vi "Numeric String to Bytes.vi"(9 "Type":T1(ring), 11 "String":string) -> (0 "error out":errorcluster, 3 "Byte Data":u8[](array[numeric]) format="%02x")   [LabVIEW 2020]
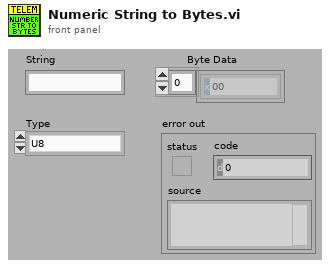
[diagram p1: front panel]
types:
  T1 = enum16{"U8", "U16", "U32", "U64", "I8", "I16", "I32", "I64"}
  T2 = cluster{"Byte Data[0]":u8, "Byte Data[1]":u8, "Byte Data[2]":u8, "Byte Data[3]":u8}
  T3 = cluster{"Byte Data[0]":u8, "Byte Data[1]":u8, "Byte Data[2]":u8, "Byte Data[3]":u8, "Byte Data[4]":u8, "Byte Data[5]":u8, "Byte Data[6]":u8, "Byte Data[7]":u8}
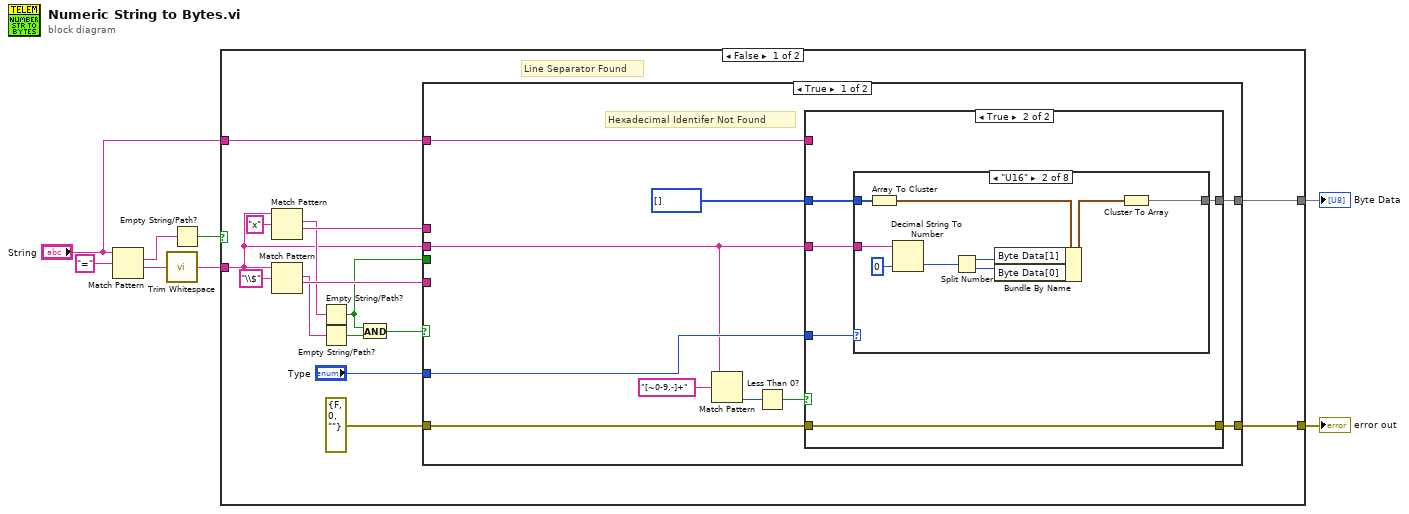
[diagram p0: block diagram]
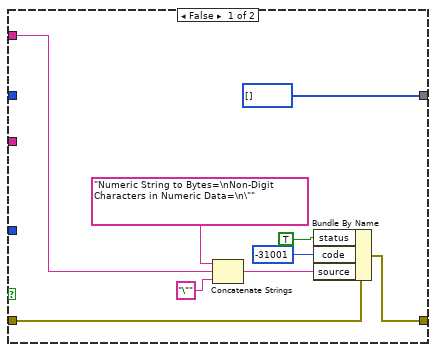
[diagram p2: hidden frame]
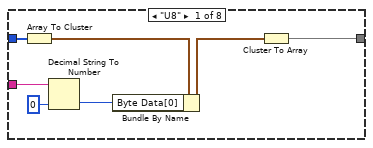
[diagram p3: hidden frame]
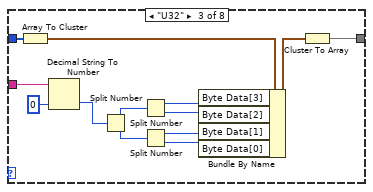
[diagram p4: hidden frame]
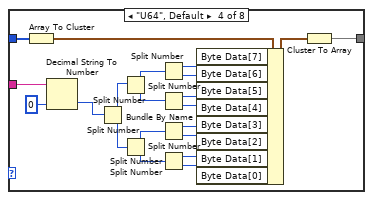
[diagram p5: hidden frame]
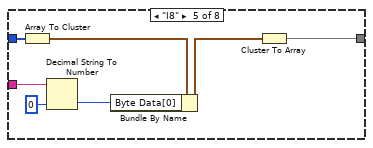
[diagram p6: hidden frame]
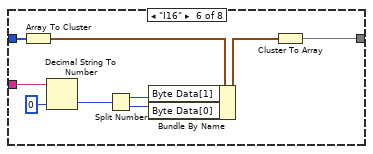
[diagram p7: hidden frame]
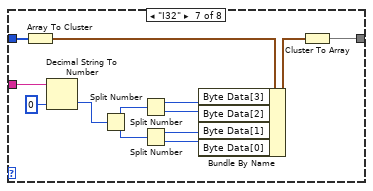
[diagram p8: hidden frame]
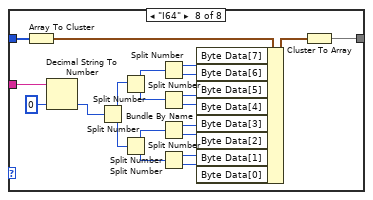
[diagram p9: hidden frame]
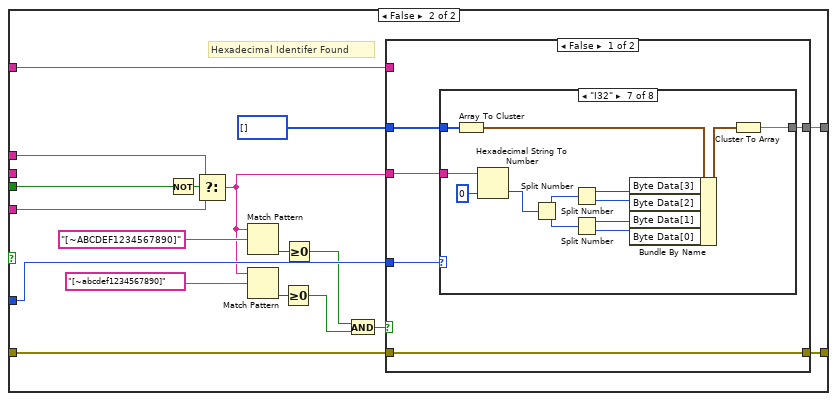
[diagram p10: hidden frame]
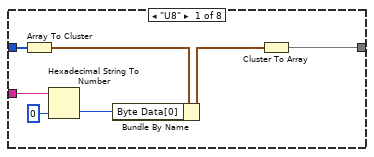
[diagram p11: hidden frame]
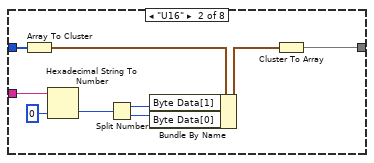
[diagram p12: hidden frame]
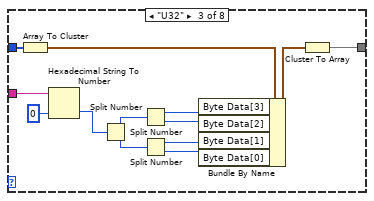
[diagram p13: hidden frame]
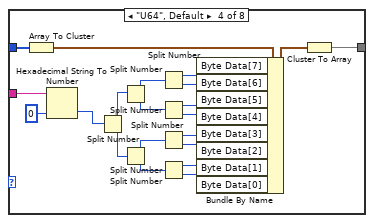
[diagram p14: hidden frame]
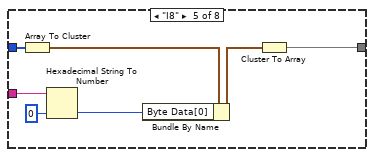
[diagram p15: hidden frame]
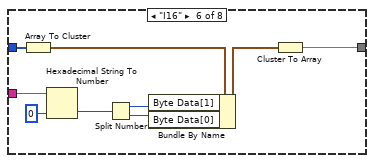
[diagram p16: hidden frame]
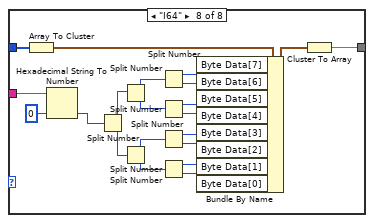
[diagram p17: hidden frame]
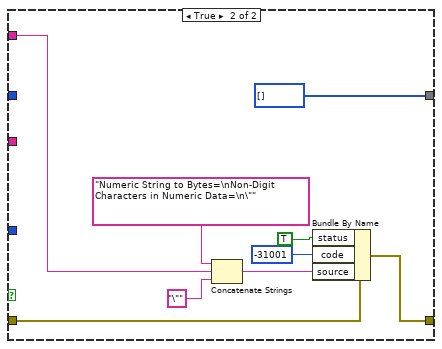
[diagram p18: hidden frame]
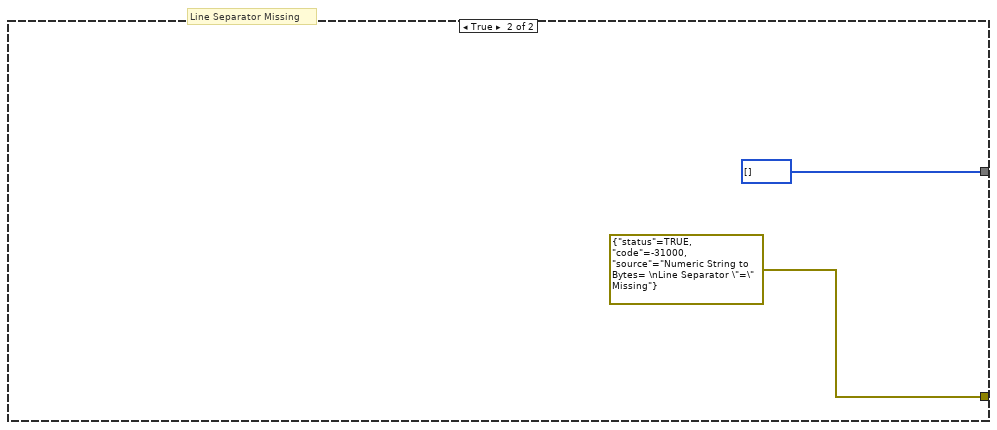
[diagram p19: hidden frame]
diagram:
  n1 = Match Pattern(string="String", regular expression="=") -> (match substring=w7:string, after substring=w6:string)  [unwired: 1 in, 2 out]
  n2 = call <vilib>:"Trim Whitespace.vi"("string"=w6) -> ("trimmed string"=w2:string)  [unwired: 1 in]
  n3 = Empty String/Path?(string/path=w7) -> (empty?=w5:bool)
  n4 = case shown="False" w5 {
    tunnel: w2 -> [w10 _]
    tunnel: [w13 u8[] [] ("Byte Data")] -> w4
    tunnel: [w11 errorcluster {"status"=TRUE, "code"=-31000, "source"="Numeric String to Bytes= \nLine Separator \"=\" Missing"} ("error out")] -> w3
    tunnel: "String" -> [w9 _]
    frame False {
      # "Line Separator Found"
      n5 = Match Pattern(string=w10, regular expression="x") -> (match substring=w19:string, after substring=w21:string)  [unwired: 1 in, 2 out]
      n6 = Match Pattern(string=w10, regular expression="\\$") -> (match substring=w18:string, after substring=w20:string)  [unwired: 1 in, 2 out]
      n7 = Empty String/Path?(string/path=w19) -> (empty?=w15:bool)
      n8 = Empty String/Path?(string/path=w18) -> (empty?=w16:bool)
      n9 = And(x=w15, y=w16) -> (x .and. y?=w17:bool)
      n10 = case shown="True" w17 {
        tunnel: w21 -> [_ w162]
        tunnel: w20 -> [_ w161]
        tunnel: w15 -> [_ w159]
        tunnel: [w31 w163] -> w13
        tunnel: w10 -> [w25 _]
        tunnel: "Type" -> [w33 w165]
        tunnel: errorcluster {"status"=FALSE, "code"=0, "source"=""} ("error out") -> [w29 w155]
        tunnel: [w30 w158] -> w11
        tunnel: w9 -> [w24 w150]
        frame True {
          # "Hexadecimal Identifer Not Found"
          n11 = Match Pattern(string=w25, regular expression="[~0-9,-]+") -> (offset past match=w27:i32)  [unwired: 1 in, 3 out]
          n12 = Less Than 0?(x=w27) -> (x < 0?=w26:bool)
          n13 = case shown="True" w26 {
            tunnel: w25 -> [_ w47]
            tunnel: w33 -> [_ w46]
            tunnel: u8[] [] ("Byte Data") -> [_ w45]
            tunnel: [u8[] [] ("Byte Data") w44] -> w31
            tunnel: [w36 w43] -> w30
            tunnel: w29 -> [w35 w43]
            tunnel: w24 -> [w34 _]
            frame False {
              n14 = Concatenate Strings("Numeric String to Bytes=\nNon-Digit Characters in Numeric Data=\n\"" ("source"), w34, "\"") -> (w37:string)
              n15 = Bundle By Name(cluster=w35, "status"=TRUE, "code"=-31001, "source"=w37) -> (w36:errorcluster)
            }
            frame True {
              n16 = case shown="\"U16\"" w46 {
                tunnel: w47 -> [w49 w57 w65 w97 w104 w113 w126 w147]
                tunnel: w45 -> [w50 w56 w68 w79 w102 w111 w124 w145]
                tunnel: [w48 w55 w69 w78 w98 w105 w114 w127] -> w44
                frame "U8" {
                  n17 = Array To Cluster(array=w50) -> (cluster=w53:cluster{"Byte Data[0]":u8})
                  n18 = Decimal String To Number(string=w49, default (0L)=u8 0 ("default (0 I32)")) -> (number=w52:u8)  [unwired: 1 in, 1 out]
                  n19 = Bundle By Name(cluster=w53, "Byte Data[0]"=w52) -> (w51:cluster{"Byte Data[0]":u8})
                  n20 = Cluster To Array(cluster=w51) -> (array=w48:u8[])
                }
                frame "U16" {
                  n21 = Array To Cluster(array=w56) -> (cluster=w62:cluster{"Byte Data[0]":u8, "Byte Data[1]":u8})
                  n22 = Decimal String To Number(string=w57, default (0L)=u16 0 ("default (0 I32)")) -> (number=w61:u16)  [unwired: 1 in, 1 out]
                  n23 = Split Number(x=w61) -> (hi(x)=w60:u8, lo(x)=w59:u8)
                  n24 = Bundle By Name(cluster=w62, "Byte Data[1]"=w60, "Byte Data[0]"=w59) -> (w58:cluster{"Byte Data[0]":u8, "Byte Data[1]":u8})
                  n25 = Cluster To Array(cluster=w58) -> (array=w55:u8[])
                }
                frame "U32" {
                  n26 = Array To Cluster(array=w68) -> (cluster=w67:T2)
                  n27 = Decimal String To Number(string=w65, default (0L)=u32 0 ("default (0 I32)")) -> (number=w64:u32)  [unwired: 1 in, 1 out]
                  n28 = Split Number(x=w64) -> (hi(x)=w75:u16, lo(x)=w76:u16)
                  n29 = Split Number(x=w75) -> (hi(x)=w74:u8, lo(x)=w73:u8)
                  n30 = Split Number(x=w76) -> (hi(x)=w72:u8, lo(x)=w71:u8)
                  n31 = Bundle By Name(cluster=w67, "Byte Data[3]"=w74, "Byte Data[2]"=w73, "Byte Data[1]"=w72, "Byte Data[0]"=w71) -> (w70:T2)
                  n32 = Cluster To Array(cluster=w70) -> (array=w69:u8[])
                }
                frame "U64", Default {
                  n33 = Array To Cluster(array=w79) -> (cluster=w95:T3)
                  n34 = Decimal String To Number(string=w97, default (0L)=u64 0 ("default (0 I32)")) -> (number=w77:u64)  [unwired: 1 in, 1 out]
                  n35 = Split Number(x=w77) -> (hi(x)=w94:u32, lo(x)=w93:u32)
                  n36 = Split Number(x=w94) -> (hi(x)=w91:u16, lo(x)=w92:u16)
                  n37 = Split Number(x=w93) -> (hi(x)=w90:u16, lo(x)=w89:u16)
                  n38 = Split Number(x=w91) -> (hi(x)=w88:u8, lo(x)=w87:u8)
                  n39 = Split Number(x=w92) -> (hi(x)=w86:u8, lo(x)=w85:u8)
                  n40 = Split Number(x=w90) -> (hi(x)=w84:u8, lo(x)=w83:u8)
                  n41 = Split Number(x=w89) -> (hi(x)=w82:u8, lo(x)=w81:u8)
                  n42 = Bundle By Name(cluster=w95, "Byte Data[7]"=w88, "Byte Data[6]"=w87, "Byte Data[5]"=w86, "Byte Data[4]"=w85, "Byte Data[3]"=w84, "Byte Data[2]"=w83, "Byte Data[1]"=w82, "Byte Data[0]"=w81) -> (w80:T3)
                  n43 = Cluster To Array(cluster=w80) -> (array=w78:u8[])
                }
                frame "I8" {
                  n44 = Array To Cluster(array=w102) -> (cluster=w101:cluster{"Byte Data[0]":u8})
                  n45 = Decimal String To Number(string=w104, default (0L)=i8 0 ("default (0 I32)")) -> (number=w100:i8)  [unwired: 1 in, 1 out]
                  n46 = Bundle By Name(cluster=w101, "Byte Data[0]"=w100) -> (w99:cluster{"Byte Data[0]":u8})
                  n47 = Cluster To Array(cluster=w99) -> (array=w98:u8[])
                }
                frame "I16" {
                  n48 = Array To Cluster(array=w111) -> (cluster=w110:cluster{"Byte Data[0]":u8, "Byte Data[1]":u8})
                  n49 = Decimal String To Number(string=w113, default (0L)=i16 0 ("default (0 I32)")) -> (number=w109:i16)  [unwired: 1 in, 1 out]
                  n50 = Split Number(x=w109) -> (hi(x)=w108:u8, lo(x)=w107:u8)
                  n51 = Bundle By Name(cluster=w110, "Byte Data[1]"=w108, "Byte Data[0]"=w107) -> (w106:cluster{"Byte Data[0]":u8, "Byte Data[1]":u8})
                  n52 = Cluster To Array(cluster=w106) -> (array=w105:u8[])
                }
                frame "I32" {
                  n53 = Array To Cluster(array=w124) -> (cluster=w123:T2)
                  n54 = Decimal String To Number(string=w126, default (0L)=0 ("default (0 I32)")) -> (number=w120:i32)  [unwired: 1 in, 1 out]
                  n55 = Split Number(x=w120) -> (hi(x)=w121:u16, lo(x)=w122:u16)
                  n56 = Split Number(x=w121) -> (hi(x)=w119:u8, lo(x)=w118:u8)
                  n57 = Split Number(x=w122) -> (hi(x)=w117:u8, lo(x)=w116:u8)
                  n58 = Bundle By Name(cluster=w123, "Byte Data[3]"=w119, "Byte Data[2]"=w118, "Byte Data[1]"=w117, "Byte Data[0]"=w116) -> (w115:T2)
                  n59 = Cluster To Array(cluster=w115) -> (array=w114:u8[])
                }
                frame "I64" {
                  n60 = Array To Cluster(array=w145) -> (cluster=w144:T3)
                  n61 = Decimal String To Number(string=w147, default (0L)=i64 0 ("default (0 I32)")) -> (number=w143:i64)  [unwired: 1 in, 1 out]
                  n62 = Split Number(x=w143) -> (hi(x)=w142:u32, lo(x)=w141:u32)
                  n63 = Split Number(x=w142) -> (hi(x)=w139:u16, lo(x)=w140:u16)
                  n64 = Split Number(x=w141) -> (hi(x)=w138:u16, lo(x)=w137:u16)
                  n65 = Split Number(x=w139) -> (hi(x)=w136:u8, lo(x)=w135:u8)
                  n66 = Split Number(x=w140) -> (hi(x)=w134:u8, lo(x)=w133:u8)
                  n67 = Split Number(x=w138) -> (hi(x)=w132:u8, lo(x)=w131:u8)
                  n68 = Split Number(x=w137) -> (hi(x)=w130:u8, lo(x)=w129:u8)
                  n69 = Bundle By Name(cluster=w144, "Byte Data[7]"=w136, "Byte Data[6]"=w135, "Byte Data[5]"=w134, "Byte Data[4]"=w133, "Byte Data[3]"=w132, "Byte Data[2]"=w131, "Byte Data[1]"=w130, "Byte Data[0]"=w129) -> (w128:T3)
                  n70 = Cluster To Array(cluster=w128) -> (array=w127:u8[])
                }
              }
            }
          }
        }
        frame False {
          # "Hexadecimal Identifer Found"
          n71 = Not(x=w159) -> (.not. x?=w160:bool)
          n72 = Select(t=w162, s=w160, f=w161) -> (s? t:f=w151:string)
          n73 = Match Pattern(string=w151, regular expression="[~ABCDEF1234567890]") -> (offset past match=w156:i32)  [unwired: 1 in, 3 out]
          n74 = Match Pattern(string=w151, regular expression="[~abcdef1234567890]") -> (offset past match=w152:i32)  [unwired: 1 in, 3 out]
          n75 = Greater Or Equal To 0?(x=w152) -> (x >= 0?=w148:bool)
          n76 = Greater Or Equal To 0?(x=w156) -> (x >= 0?=w154:bool)
          n77 = And(x=w154, y=w148) -> (x .and. y?=w153:bool)
          n78 = case shown="False" w153 {
            tunnel: w165 -> [w170 _]
            tunnel: u8[] [] ("Byte Data") -> [w169 _]
            tunnel: [w168 u8[] [] ("Byte Data")] -> w163
            tunnel: w151 -> [w167 _]
            tunnel: [w166 w277] -> w158
            tunnel: w155 -> [w166 w278]
            tunnel: w150 -> [_ w271]
            frame False {
              n79 = case shown="\"I32\"" w170 {
                tunnel: w167 -> [w172 w180 w188 w220 w227 w236 w249 w270]
                tunnel: w169 -> [w173 w179 w191 w202 w225 w234 w247 w268]
                tunnel: [w171 w178 w192 w201 w222 w228 w237 w250] -> w168
                frame "U8" {
                  n80 = Array To Cluster(array=w173) -> (cluster=w176:cluster{"Byte Data[0]":u8})
                  n81 = Hexadecimal String To Number(string=w172, default (0uL)=u8 0 ("default (0 I32)")) -> (number=w175:u8)  [unwired: 1 in, 1 out]
                  n82 = Bundle By Name(cluster=w176, "Byte Data[0]"=w175) -> (w174:cluster{"Byte Data[0]":u8})
                  n83 = Cluster To Array(cluster=w174) -> (array=w171:u8[])
                }
                frame "U16" {
                  n84 = Array To Cluster(array=w179) -> (cluster=w185:cluster{"Byte Data[0]":u8, "Byte Data[1]":u8})
                  n85 = Hexadecimal String To Number(string=w180, default (0uL)=u16 0 ("default (0 I32)")) -> (number=w184:u16)  [unwired: 1 in, 1 out]
                  n86 = Split Number(x=w184) -> (hi(x)=w183:u8, lo(x)=w182:u8)
                  n87 = Bundle By Name(cluster=w185, "Byte Data[1]"=w183, "Byte Data[0]"=w182) -> (w181:cluster{"Byte Data[0]":u8, "Byte Data[1]":u8})
                  n88 = Cluster To Array(cluster=w181) -> (array=w178:u8[])
                }
                frame "U32" {
                  n89 = Array To Cluster(array=w191) -> (cluster=w190:T2)
                  n90 = Hexadecimal String To Number(string=w188, default (0uL)=u32 0 ("default (0 I32)")) -> (number=w187:u32)  [unwired: 1 in, 1 out]
                  n91 = Split Number(x=w187) -> (hi(x)=w198:u16, lo(x)=w199:u16)
                  n92 = Split Number(x=w198) -> (hi(x)=w197:u8, lo(x)=w196:u8)
                  n93 = Split Number(x=w199) -> (hi(x)=w195:u8, lo(x)=w194:u8)
                  n94 = Bundle By Name(cluster=w190, "Byte Data[3]"=w197, "Byte Data[2]"=w196, "Byte Data[1]"=w195, "Byte Data[0]"=w194) -> (w193:T2)
                  n95 = Cluster To Array(cluster=w193) -> (array=w192:u8[])
                }
                frame "U64", Default {
                  n96 = Array To Cluster(array=w202) -> (cluster=w218:T3)
                  n97 = Hexadecimal String To Number(string=w220, default (0uL)=u64 0 ("default (0 I32)")) -> (number=w200:u64)  [unwired: 1 in, 1 out]
                  n98 = Split Number(x=w200) -> (hi(x)=w217:u32, lo(x)=w216:u32)
                  n99 = Split Number(x=w217) -> (hi(x)=w214:u16, lo(x)=w215:u16)
                  n100 = Split Number(x=w216) -> (hi(x)=w213:u16, lo(x)=w212:u16)
                  n101 = Split Number(x=w214) -> (hi(x)=w211:u8, lo(x)=w210:u8)
                  n102 = Split Number(x=w215) -> (hi(x)=w209:u8, lo(x)=w208:u8)
                  n103 = Split Number(x=w213) -> (hi(x)=w207:u8, lo(x)=w206:u8)
                  n104 = Split Number(x=w212) -> (hi(x)=w205:u8, lo(x)=w204:u8)
                  n105 = Bundle By Name(cluster=w218, "Byte Data[7]"=w211, "Byte Data[6]"=w210, "Byte Data[5]"=w209, "Byte Data[4]"=w208, "Byte Data[3]"=w207, "Byte Data[2]"=w206, "Byte Data[1]"=w205, "Byte Data[0]"=w204) -> (w203:T3)
                  n106 = Cluster To Array(cluster=w203) -> (array=w201:u8[])
                }
                frame "I8" {
                  n107 = Array To Cluster(array=w225) -> (cluster=w224:cluster{"Byte Data[0]":u8})
                  n108 = Hexadecimal String To Number(string=w227, default (0uL)=i8 0 ("default (0 I32)")) -> (number=w221:i8)  [unwired: 1 in, 1 out]
                  n109 = Bundle By Name(cluster=w224, "Byte Data[0]"=w221) -> (w223:cluster{"Byte Data[0]":u8})
                  n110 = Cluster To Array(cluster=w223) -> (array=w222:u8[])
                }
                frame "I16" {
                  n111 = Array To Cluster(array=w234) -> (cluster=w233:cluster{"Byte Data[0]":u8, "Byte Data[1]":u8})
                  n112 = Hexadecimal String To Number(string=w236, default (0uL)=i16 0 ("default (0 I32)")) -> (number=w232:i16)  [unwired: 1 in, 1 out]
                  n113 = Split Number(x=w232) -> (hi(x)=w231:u8, lo(x)=w230:u8)
                  n114 = Bundle By Name(cluster=w233, "Byte Data[1]"=w231, "Byte Data[0]"=w230) -> (w229:cluster{"Byte Data[0]":u8, "Byte Data[1]":u8})
                  n115 = Cluster To Array(cluster=w229) -> (array=w228:u8[])
                }
                frame "I32" {
                  n116 = Array To Cluster(array=w247) -> (cluster=w246:T2)
                  n117 = Hexadecimal String To Number(string=w249, default (0uL)=0 ("default (0 I32)")) -> (number=w243:i32)  [unwired: 1 in, 1 out]
                  n118 = Split Number(x=w243) -> (hi(x)=w244:u16, lo(x)=w245:u16)
                  n119 = Split Number(x=w244) -> (hi(x)=w242:u8, lo(x)=w241:u8)
                  n120 = Split Number(x=w245) -> (hi(x)=w240:u8, lo(x)=w239:u8)
                  n121 = Bundle By Name(cluster=w246, "Byte Data[3]"=w242, "Byte Data[2]"=w241, "Byte Data[1]"=w240, "Byte Data[0]"=w239) -> (w238:T2)
                  n122 = Cluster To Array(cluster=w238) -> (array=w237:u8[])
                }
                frame "I64" {
                  n123 = Array To Cluster(array=w268) -> (cluster=w267:T3)
                  n124 = Hexadecimal String To Number(string=w270, default (0uL)=i64 0 ("default (0 I32)")) -> (number=w266:i64)  [unwired: 1 in, 1 out]
                  n125 = Split Number(x=w266) -> (hi(x)=w265:u32, lo(x)=w264:u32)
                  n126 = Split Number(x=w265) -> (hi(x)=w262:u16, lo(x)=w263:u16)
                  n127 = Split Number(x=w264) -> (hi(x)=w261:u16, lo(x)=w260:u16)
                  n128 = Split Number(x=w262) -> (hi(x)=w259:u8, lo(x)=w258:u8)
                  n129 = Split Number(x=w263) -> (hi(x)=w257:u8, lo(x)=w256:u8)
                  n130 = Split Number(x=w261) -> (hi(x)=w255:u8, lo(x)=w254:u8)
                  n131 = Split Number(x=w260) -> (hi(x)=w253:u8, lo(x)=w252:u8)
                  n132 = Bundle By Name(cluster=w267, "Byte Data[7]"=w259, "Byte Data[6]"=w258, "Byte Data[5]"=w257, "Byte Data[4]"=w256, "Byte Data[3]"=w255, "Byte Data[2]"=w254, "Byte Data[1]"=w253, "Byte Data[0]"=w252) -> (w251:T3)
                  n133 = Cluster To Array(cluster=w251) -> (array=w250:u8[])
                }
              }
            }
            frame True {
              n134 = Concatenate Strings("Numeric String to Bytes=\nNon-Digit Characters in Numeric Data=\n\"" ("source"), w271, "\"") -> (w272:string)
              n135 = Bundle By Name(cluster=w278, "status"=TRUE, "code"=-31001, "source"=w272) -> (w277:errorcluster)
            }
          }
        }
      }
    }
    frame True {
      # "Line Separator Missing"
    }
  }
  "error out" <- w3
  "Byte Data" <- w4
